vi "Get Setpoint.vi"(8 "error in (no error)":errorcluster, 10 "Output (0:Sample Heater)":u16(ring) items=["Sample Heater", "Warm-up Heater (Output 1)"], 11 "VISA resource name":refnum<visa-resource-name>) -> (0 "error out":errorcluster, 2 "Setpoint (0.00000E+0)":dbl min=0.0 max=100000000.0 step=1e-06 format="%^.5e", 3 "VISA resource name out":refnum<visa-resource-name>)   [LabVIEW 2018, in "Lake Shore 372.lvlib"]
doc: "Queries the value of the temperature control setpoint."
uses:
  Lake Shore 372.lvlib
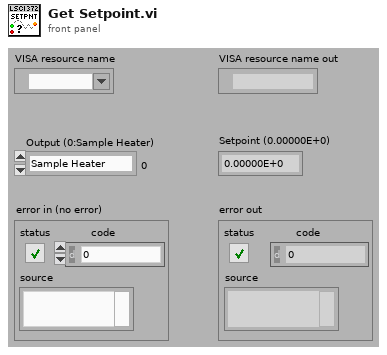
[diagram p1: front panel]
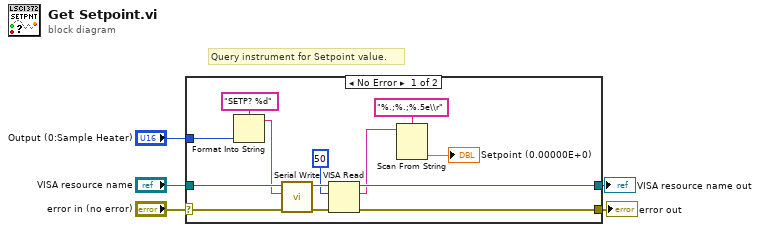
[diagram p0: block diagram]
diagram:
  # "Query instrument for Setpoint value."
  n1 = case shown="No Error" "error in (no error)" {
    selector: "error in (no error)" -> [w6 w19]
    tunnel: "VISA resource name" -> [w13 w20]
    tunnel: [w12 w20] -> w4
    tunnel: [w11 w19] -> w3
    tunnel: "Output (0:Sample Heater)" -> [w8 _]
    frame No Error {
      n2 = Format Into String(format string="SETP? %d", w8) -> (resulting string=w7:string)  [unwired: 2 in, 1 out]
      n3 = call "Serial Write.vi"("error in (no error)"=w6, "Write Buffer (\"\")"=w7, "VISA resource name"=w13) -> ("error out"=w15:errorcluster, "VISA resource name out"=w16:refnum<visa-resource-name>)  [unwired: 6 in, 1 out]
      n4 = VISA Read(VISA resource name=w16, byte count=50, error in (no error)=w15) -> (VISA resource name out=w12:refnum<visa-resource-name>, read buffer=w10:string, error out=w11:errorcluster)  [unwired: 1 out]
      n5 = Scan From String(format string="%.;%.;%.5e\\r", input string=w10) -> (output 1=→"Setpoint (0.00000E+0)":dbl)  [unwired: 3 in, 3 out]
    }
    frame Error {
    }
  }
  "error out" <- w3
  "VISA resource name out" <- w4
